vi "SendListToDAQ.vi"(8 "error in":errorcluster, 10 "Input":u32[][](array[numeric]), 11 "Refnum in":refnum<k21>) -> (0 "error out":errorcluster, 3 "Refnum out":refnum<k21>)   [LabVIEW 2017, in "AODControl.lvlib"]
uses:
  AODControl.lvlib
  <vilib>/DAQmx/write.llb/DAQmx Write (Digital 2D U32 NChan NSamp).vi
  <vilib>/DAQmx/miscellaneous.llb/DAQmx Fill In Error Info.vi
  <resource>/objmgr/daqmx.rc
panel:
  out "Input 2":u32[][](array[numeric])
  out "size(s)":u32
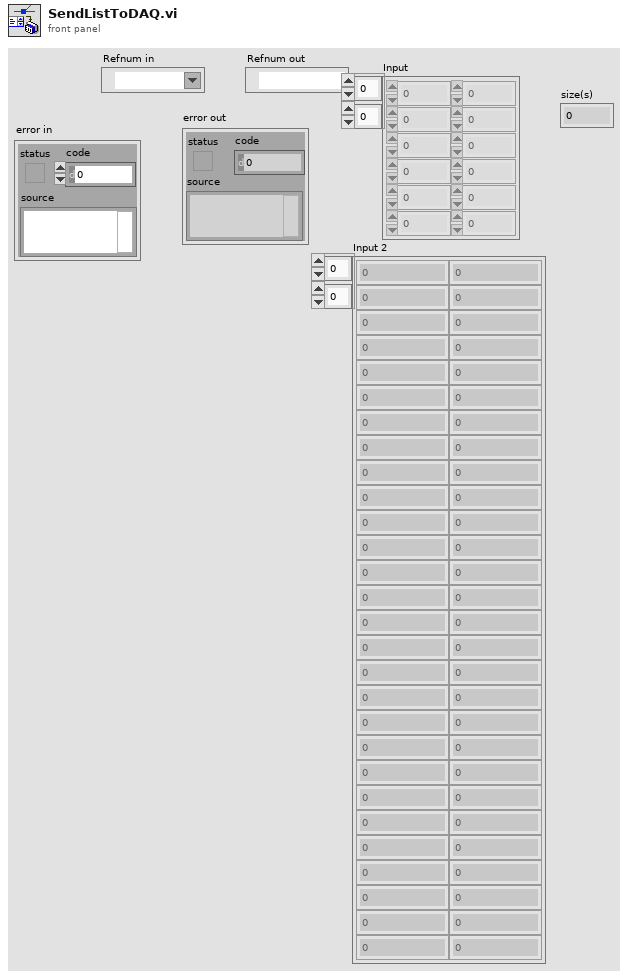
[diagram p1: front panel]
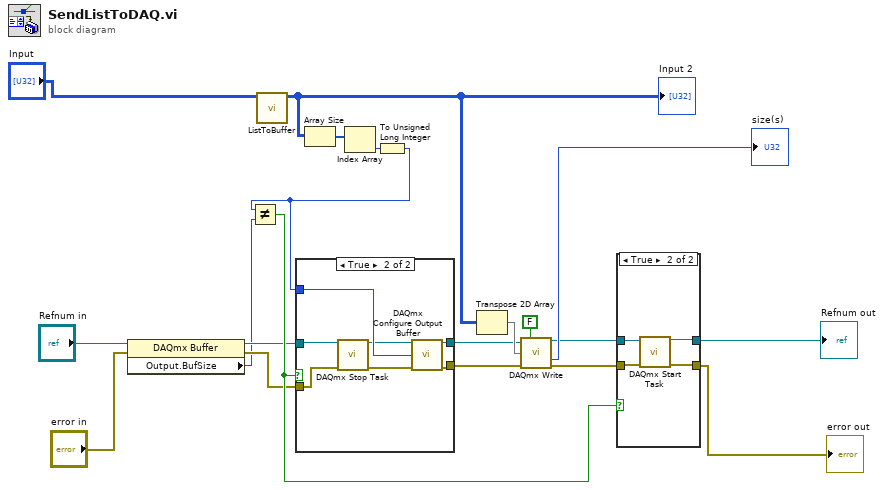
[diagram p0: block diagram]
diagram:
  n1 = property class="DAQmx Buffer"(reference="Refnum in", error in="error in") -> (reference out=w4:refnum<k21>, error out=w2:errorcluster, "Output.BufSize"=w1:u32)
  n2 = call "ListToBuffer.vi"("Input"="Input") -> ("Array"=w17:u32[][])  [unwired: 10 in]
  "Input 2" <- w17
  n3 = Array Size(array=w17) -> (size(s)=w16:i32[])
  n4 = Index Array(array=w16) -> (element=w12:i32)  [unwired: 1 in]
  n5 = To Unsigned Long Integer(number=w12) -> (unsigned 32bit integer=w13:u32)
  n6 = Not Equal?(x=w13, y=w1) -> (x != y?=w6:bool)
  n7 = case shown="True" w6 {
    tunnel: w4 -> [w22 w27]
    tunnel: w2 -> [w21 w26]
    tunnel: w13 -> [_ w29]
    tunnel: [w22 w23] -> w15
    tunnel: [w21 w24] -> w14
    frame False {
    }
    frame True {
      n8 = call <vilib>:"DAQmx Stop Task.vi"("task/channels in"=w27, "error in"=w26) -> ("task out"=w28:refnum<k21>, "error out"=w25:errorcluster)  [unwired: 12 in]
      n9 = call <vilib>:"DAQmx Configure Output Buffer.vi"("task/channels in"=w28, "buffer size (in samples per channel)"=w29, "error in"=w25) -> ("task out"=w23:refnum<k21>, "error out"=w24:errorcluster)  [unwired: 11 in]
    }
  }
  n10 = Transpose 2D Array(2D array=w17) -> (transposed array=w18:u32[][])
  n11 = call-poly <vilib>:"DAQmx Write.vi"("task/channels in"=w15, "auto start"=FALSE, "data"=w18, "error in"=w14) -> ("task out"=w8:refnum<k21>, "number of samples written per channel"=→"size(s)":u32, "error out"=w10:errorcluster)  [unwired: 9 in]
  n12 = case shown="True" w6 {
    tunnel: w8 -> [w31 w35]
    tunnel: w10 -> [w30 w34]
    tunnel: [w31 w32] -> w7
    tunnel: [w30 w33] -> w9
    frame False {
    }
    frame True {
      n13 = call <vilib>:"DAQmx Start Task.vi"("task/channels in"=w35, "error in"=w34) -> ("task out"=w32:refnum<k21>, "error out"=w33:errorcluster)  [unwired: 12 in]
    }
  }
  "Refnum out" <- w7
  "error out" <- w9
